vi "EventsLogRef Global.vi"() -> ()   [LabVIEW 2019, in "EventLog.lvlib" / "EventLog.lvclass"]
uses:
  EventLog.lvclass
panel:
  in  "EventLogRef":refnum<class "EventLog.lvclass">
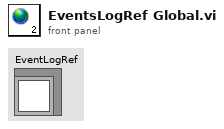
[diagram p1: front panel]
diagram:
